vi "Teleop.vi"(10 "Match Info":T1={"Autonomous Elapsed Seconds"=0.0, "TeleOp Elapsed Seconds"=0.0, "Disabled Elapsed Seconds"=0.0, "Visited Autonomous"=FALSE, "Visited TeleOp"=FALSE, "Visited Disabled"=FALSE, "Autonomous Settings"={"Autonomous Style"=enum."Independent", "VI Refnum"=refnum}}, 11 "Call Context":T2) -> ()   [LabVIEW 2019]
doc: "This VI is called for each enabled TeleOp packet received from the DS. It is typically used to read from joysticks and other inputs and update I/O or setpoints for timed control loops. It should complete and return within 20 milliseconds or risk missing DS packets."
uses:
  <vilib>/Rock Robotics/WPI/DriverStation/WPI_DriverStationDerivedRobotMode.ctl
  <vilib>/Rock Robotics/WPI/DriverStation/WPI_DriverStationMatch Info.ctl
  Framework/Robot Global Data.vi
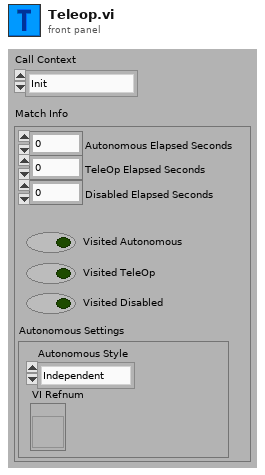
[diagram p1: front panel]
types:
  T1 = typedef "WPI_DriverStationMatch Info.ctl" = cluster{"Autonomous Elapsed Seconds":dbl, "TeleOp Elapsed Seconds":dbl, "Disabled Elapsed Seconds":dbl, "Visited Autonomous":bool, "Visited TeleOp":bool, "Visited Disabled":bool, "Autonomous Settings":cluster{"Autonomous Style":enum16{"Iterative", "Independent"}, "VI Refnum":refnum<vi>}}
  T2 = typedef "WPI_DriverStationDerivedRobotMode.ctl" = enum16{"Init", "Execute", "Stop"}
  T3 = typedef "Command Status Info.ctl" = cluster{"Name":string, "Status":T4, "notifier out":T5}
  T4 = typedef "Completion Status.ctl" = enum16{"Successful", "Aborted", "Incomplete"}
  T5 = typedef "Completion Notifier.ctl" = refnum<notifier>
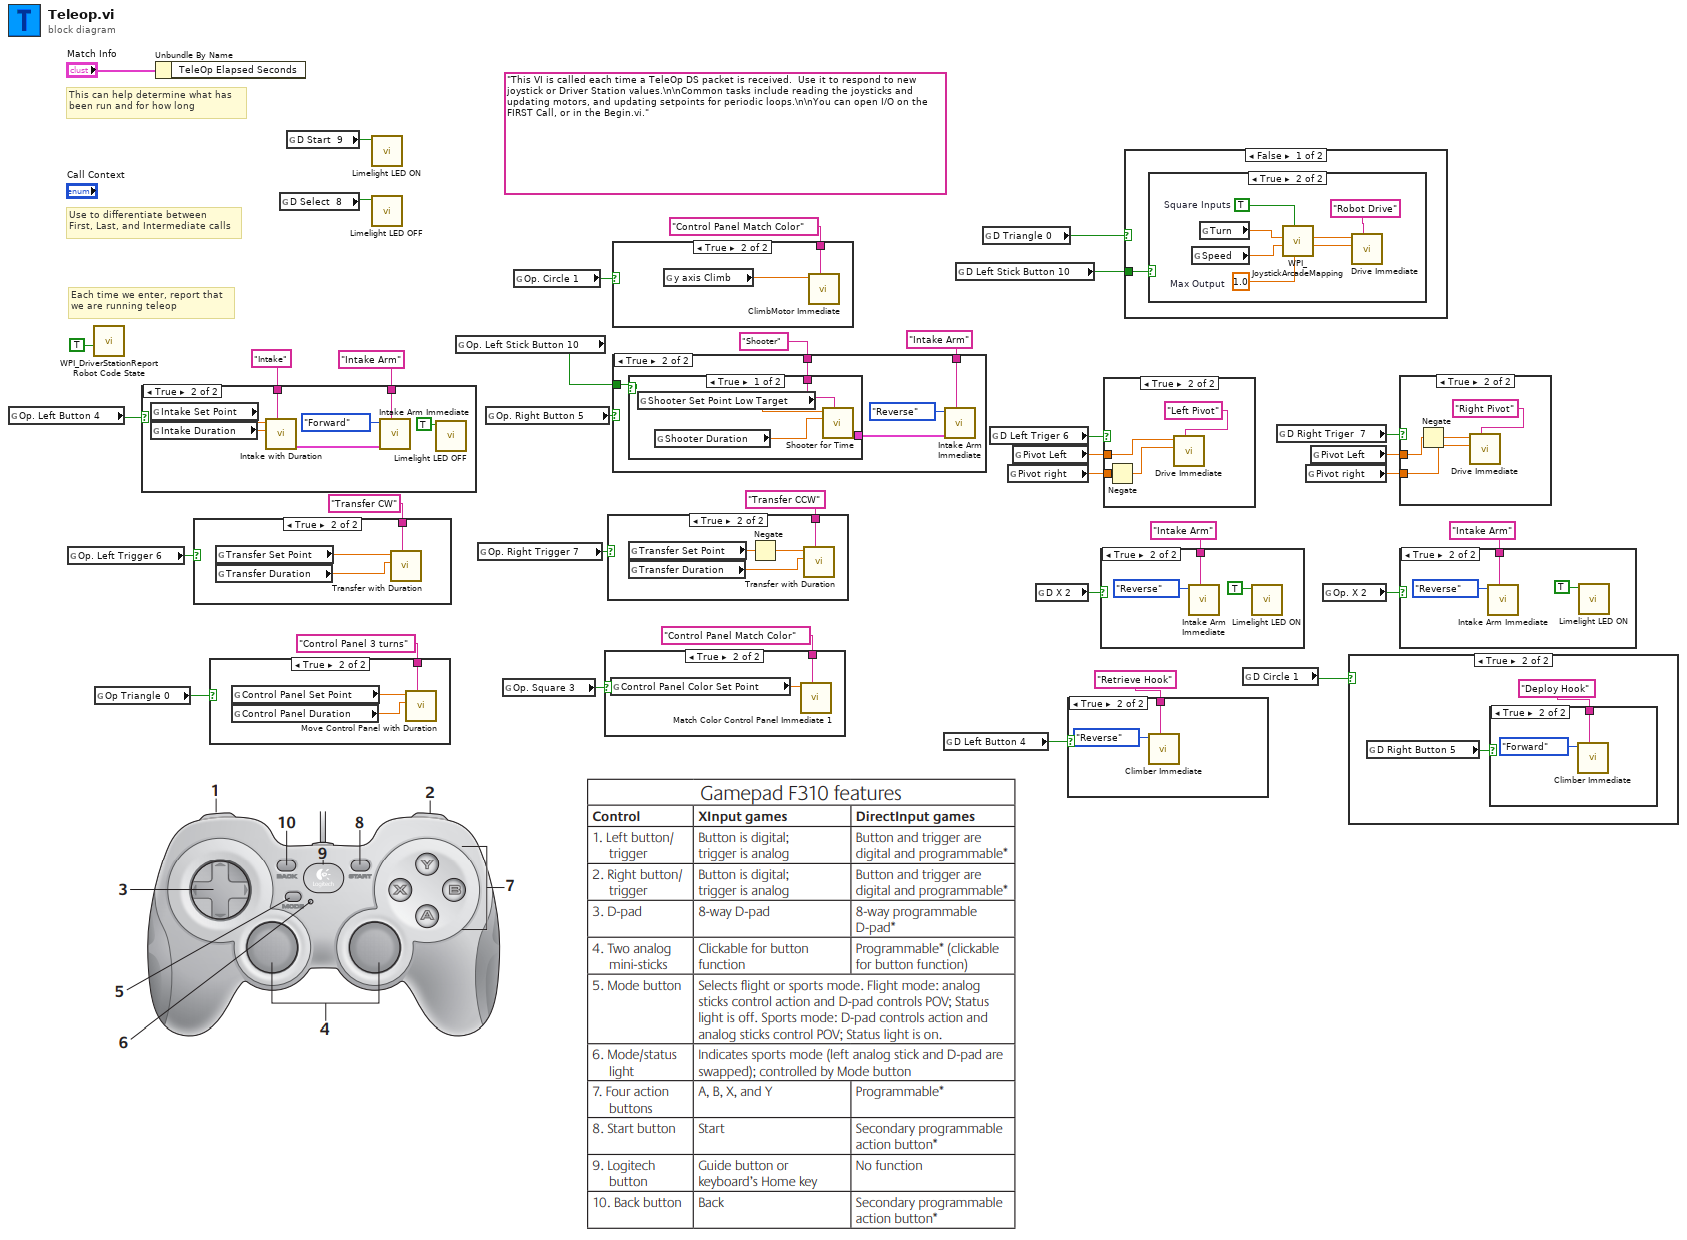
[diagram p0: block diagram]
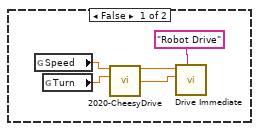
[diagram p7: hidden frame]
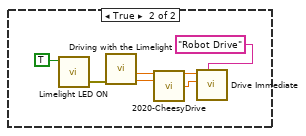
[diagram p8: hidden frame]
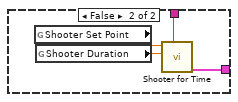
[diagram p17: hidden frame]
diagram:
  (unwired) "This VI is called each time a TeleOp DS packet is received.  Use it to respond to new joystick or Driver Station values.\n\nCommon tasks include reading the joysticks and updating motors, and updating setpoints for periodic loops.\n\nYou can open I/O on the FIRST Call, or in the Begin.vi."
  # "Each time we enter, report that\nwe are running teleop"
  # "Use to differentiate between\nFirst, Last, and Intermediate calls"
  # "This can help determine what has\nbeen run and for how long"
  n1 = global read "Robot Global Data.vi" "Op. Left Button 4"() -> (w34:bool)
  n2 = global read "Robot Global Data.vi" "Op. Left Trigger 6"() -> (w28:bool)
  n3 = call <vilib>:"WPI_DriverStationReport Robot Code State.vi"("TeleOp"=TRUE ("Autonomous")) -> ()  [unwired: 10 in, 1 out]
  n4 = global read "Robot Global Data.vi" "Op Triangle 0"() -> (w21:bool)
  n5 = case shown="True" w34 {
    tunnel: "Intake" ("refnum name") -> [_ w43]
    tunnel: "Intake Arm" ("refnum name") -> [_ w39]
    frame False {
    }
    frame True {
      n6 = global read "Robot Global Data.vi" "Intake Set Point"() -> (w42:dbl)
      n7 = global read "Robot Global Data.vi" "Intake Duration"() -> (w41:dbl)
      n8 = call "Intake with Duration.vi"("Description"=w43, "Duration (s)"=w41, "Setpoint"=w42) -> ("Command Info Out"=w38:T3)  [unwired: 8 in]
      n9 = call "Intake Arm Immediate.vi"("Description"=w39, "Command Info In"=w38, "Relay Value"=enum16{"Off", "On", "Forward", "Reverse"}."Forward") -> ()  [unwired: 8 in, 1 out]
      n10 = call "Limelight LED OFF.vi"("D Select  8"=TRUE) -> ()  [unwired: 11 in]
    }
  }
  n11 = Unbundle By Name("Match Info") -> ()  [unwired: 1 out]
  n12 = case shown="True" w28 {
    tunnel: "Transfer CW" ("refnum name") -> [_ w46]
    frame False {
    }
    frame True {
      n13 = global read "Robot Global Data.vi" "Transfer Set Point"() -> (w45:dbl)
      n14 = global read "Robot Global Data.vi" "Transfer Duration"() -> (w44:dbl)
      n15 = call "Transfer with Duration.vi"("Description"=w46, "Duration (s)"=w44, "Setpoint"=w45) -> ()  [unwired: 8 in, 1 out]
    }
  }
  n16 = case shown="True" w21 {
    tunnel: "Control Panel 3 turns" ("refnum name") -> [_ w49]
    frame False {
    }
    frame True {
      n17 = global read "Robot Global Data.vi" "Control Panel Set Point"() -> (w48:dbl)
      n18 = global read "Robot Global Data.vi" "Control Panel Duration"() -> (w47:dbl)
      n19 = call "Move Control Panel with Duration.vi"("Description"=w49, "Duration (s)"=w47, "Setpoint"=w48) -> ()  [unwired: 8 in, 1 out]
    }
  }
  n20 = global read "Robot Global Data.vi" "D Select  8"() -> (w2:bool)
  n21 = global read "Robot Global Data.vi" "D Start  9"() -> (w3:bool)
  n22 = call "Limelight LED ON.vi"("D Start  9"=w3) -> ()  [unwired: 10 in, 1 out]
  n23 = call "Limelight LED OFF.vi"("D Select  8"=w2) -> ()  [unwired: 11 in]
  n24 = global read "Robot Global Data.vi" "Op. Left Stick Button 10"() -> (w4:bool)
  n25 = global read "Robot Global Data.vi" "Op. Right Trigger 7"() -> (w29:bool)
  n26 = global read "Robot Global Data.vi" "Op. Right Button 5"() -> (w30:bool)
  n27 = global read "Robot Global Data.vi" "Op. Square 3"() -> (w18:bool)
  n28 = global read "Robot Global Data.vi" "Op. Circle 1"() -> (w6:bool)
  n29 = case shown="True" w18 {
    tunnel: "Control Panel Match Color" ("refnum name") -> [_ w51]
    frame False {
    }
    frame True {
      n30 = global read "Robot Global Data.vi" "Control Panel Color Set Point"() -> (w50:dbl)
      n31 = call "Match Color Control Panel Immediate 1.vi"("Description"=w51, "Setpoint"=w50) -> ()  [unwired: 9 in, 1 out]
    }
  }
  n32 = case shown="True" w29 {
    tunnel: "Transfer CCW" ("refnum name") -> [_ w55]
    frame False {
    }
    frame True {
      n33 = global read "Robot Global Data.vi" "Transfer Set Point"() -> (w53:dbl)
      n34 = global read "Robot Global Data.vi" "Transfer Duration"() -> (w52:dbl)
      n35 = Negate(x=w53) -> (-x=w54:dbl)
      n36 = call "Transfer with Duration.vi"("Description"=w55, "Duration (s)"=w52, "Setpoint"=w54) -> ()  [unwired: 8 in, 1 out]
    }
  }
  n37 = case shown="True" w6 {
    tunnel: "Control Panel Match Color" ("refnum name") -> [_ w57]
    frame False {
    }
    frame True {
      n38 = global read "Robot Global Data.vi" "y axis Climb"() -> (w56:dbl)
      n39 = call "ClimbMotor Immediate.vi"("Description"=w57, "Setpoint"=w56) -> ()  [unwired: 9 in, 1 out]
    }
  }
  n40 = case shown="True" w30 {
    tunnel: "Shooter" ("refnum name") -> [_ w62]
    tunnel: "Intake Arm" ("refnum name") -> [_ w60]
    tunnel: w4 -> [_ w58]
    frame False {
    }
    frame True {
      n41 = case shown="True" w58 {
        tunnel: w62 -> [w66 w70]
        tunnel: [w63 w67] -> w59
        frame True {
          n42 = global read "Robot Global Data.vi" "Shooter Set Point Low Target"() -> (w65:dbl)
          n43 = global read "Robot Global Data.vi" "Shooter Duration"() -> (w64:dbl)
          n44 = call "Shooter for Time.vi"("Description"=w66, "Duration (s)"=w64, "Setpoint"=w65) -> ("Command Info Out"=w63:T3)  [unwired: 8 in]
        }
        frame False {
          n45 = global read "Robot Global Data.vi" "Shooter Set Point"() -> (w69:dbl)
          n46 = global read "Robot Global Data.vi" "Shooter Duration"() -> (w68:dbl)
          n47 = call "Shooter for Time.vi"("Description"=w70, "Duration (s)"=w68, "Setpoint"=w69) -> ("Command Info Out"=w67:T3)  [unwired: 8 in]
        }
      }
      n48 = call "Intake Arm Immediate.vi"("Description"=w60, "Command Info In"=w59, "Relay Value"=enum16{"Off", "On", "Forward", "Reverse"}."Reverse") -> ()  [unwired: 8 in, 1 out]
    }
  }
  n49 = global read "Robot Global Data.vi" "D Left Button 4"() -> (w11:bool)
  n50 = global read "Robot Global Data.vi" "D Left Stick Button 10"() -> (w1:bool)
  n51 = global read "Robot Global Data.vi" "D Triangle 0"() -> (w12:bool)
  n52 = global read "Robot Global Data.vi" "D Left Triger 6"() -> (w26:bool)
  n53 = global read "Robot Global Data.vi" "Pivot right"() -> (w15:dbl)
  n54 = global read "Robot Global Data.vi" "Pivot Left"() -> (w16:dbl)
  n55 = global read "Robot Global Data.vi" "D X 2"() -> (w19:bool)
  n56 = case shown="True" w11 {
    tunnel: "Retrieve Hook" ("refnum name") -> [_ w71]
    frame False {
    }
    frame True {
      n57 = call "Climber Immediate.vi"("Description"=w71, "Value"=enum16{"Off", "On", "Forward", "Reverse"}."Reverse" ("Relay Value")) -> ()  [unwired: 9 in, 1 out]
    }
  }
  n58 = case shown="True" w19 {
    tunnel: "Intake Arm" ("refnum name") -> [_ w74]
    frame False {
    }
    frame True {
      n59 = call "Intake Arm Immediate.vi"("Description"=w74, "Relay Value"=enum16{"Off", "On", "Forward", "Reverse"}."Reverse") -> ()  [unwired: 9 in, 1 out]
      n60 = call "Limelight LED ON.vi"("D Start  9"=TRUE) -> ()  [unwired: 10 in, 1 out]
    }
  }
  n61 = case shown="True" w26 {
    tunnel: w16 -> [_ w78]
    tunnel: w15 -> [_ w77]
    frame False {
    }
    frame True {
      n62 = Negate(x=w77) -> (-x=w76:dbl)
      n63 = call "Drive Immediate.vi"("Description"="Left Pivot", "Right Setpoint"=w76, "Left Setpoint"=w78) -> ()  [unwired: 8 in, 1 out]
    }
  }
  n64 = case shown="False" w12 {
    tunnel: w1 -> [w80 _]
    frame False {
      n65 = case shown="True" w80 {
        frame False {
          n66 = global read "Robot Global Data.vi" "Speed"() -> (w82:dbl)
          n67 = global read "Robot Global Data.vi" "Turn"() -> (w83:dbl)
          n68 = call "2020-CheesyDrive.vi"("Throttle"=w82, "Wheel"=w83) -> ("Left PWM"=w84:dbl, "Right PWM"=w85:dbl)  [unwired: 12 in]
          n69 = call "Drive Immediate.vi"("Description"="Robot Drive", "Right Setpoint"=w85, "Left Setpoint"=w84) -> ()  [unwired: 8 in, 1 out]
        }
        frame True {
          w88 = 1.0  # Max Output
          w89 = TRUE  # Square Inputs
          n70 = global read "Robot Global Data.vi" "Speed"() -> (w90:dbl)
          n71 = global read "Robot Global Data.vi" "Turn"() -> (w91:dbl)
          n72 = call <vilib>:"WPI_JoystickArcadeMapping.vi"("Max Output"=w88, "Square Inputs"=w89, "Y axis value"=w90, "X axis value"=w91) -> ("Right Motor Value"=w86:dbl, "Left Motor Value"=w87:dbl)  [unwired: 6 in]
          n73 = call "Drive Immediate.vi"("Description"="Robot Drive", "Right Setpoint"=w86, "Left Setpoint"=w87) -> ()  [unwired: 8 in, 1 out]
        }
      }
    }
    frame True {
      n74 = call "Limelight LED ON.vi"("D Start  9"=TRUE) -> ("error out"=w94:errorcluster)  [unwired: 10 in]
      n75 = call "Driving with the Limelight.vi"("error in (no error)"=w94) -> ("TurnCommand"=w95:dbl, "SpeedCommand"=w96:dbl)  [unwired: 8 in, 1 out]
      n76 = call "2020-CheesyDrive.vi"("Throttle"=w96, "Wheel"=w95) -> ("Left PWM"=w98:dbl, "Right PWM"=w99:dbl)  [unwired: 12 in]
      n77 = call "Drive Immediate.vi"("Description"="Robot Drive", "Right Setpoint"=w99, "Left Setpoint"=w98) -> ()  [unwired: 8 in, 1 out]
    }
  }
  n78 = global read "Robot Global Data.vi" "D Circle 1"() -> (w5:bool)
  n79 = global read "Robot Global Data.vi" "D Right Triger  7"() -> (w25:bool)
  n80 = global read "Robot Global Data.vi" "Pivot right"() -> (w13:dbl)
  n81 = global read "Robot Global Data.vi" "Pivot Left"() -> (w14:dbl)
  n82 = global read "Robot Global Data.vi" "Op. X 2"() -> (w9:bool)
  n83 = case shown="True" w5 {
    frame False {
    }
    frame True {
      n84 = global read "Robot Global Data.vi" "D Right Button 5"() -> (w100:bool)
      n85 = case shown="True" w100 {
        tunnel: "Deploy Hook" ("refnum name") -> [_ w102]
        frame False {
        }
        frame True {
          n86 = call "Climber Immediate.vi"("Description"=w102, "Value"=enum16{"Off", "On", "Forward", "Reverse"}."Forward" ("Relay Value")) -> ()  [unwired: 9 in, 1 out]
        }
      }
    }
  }
  n87 = case shown="True" w25 {
    tunnel: w14 -> [_ w106]
    tunnel: w13 -> [_ w105]
    frame False {
    }
    frame True {
      n88 = Negate(x=w106) -> (-x=w104:dbl)
      n89 = call "Drive Immediate.vi"("Description"="Right Pivot", "Right Setpoint"=w105, "Left Setpoint"=w104) -> ()  [unwired: 8 in, 1 out]
    }
  }
  n90 = case shown="True" w9 {
    tunnel: "Intake Arm" ("refnum name") -> [_ w109]
    frame False {
    }
    frame True {
      n91 = call "Intake Arm Immediate.vi"("Description"=w109, "Relay Value"=enum16{"Off", "On", "Forward", "Reverse"}."Reverse") -> ()  [unwired: 9 in, 1 out]
      n92 = call "Limelight LED ON.vi"("D Start  9"=TRUE) -> ()  [unwired: 10 in, 1 out]
    }
  }
